vi "CLD 2 Elapsed Time Express FGV Exercise.vi"(7 "Express Timer FGV Enum":enum16{"Reset", "Read Status", "Set Auto Reset"}(ring), 8 "error in (no error)":errorcluster, 9 "Auto Reset (F)":bool, 11 "Time Target (s)":dbl=7.0) -> (0 "error out":errorcluster, 2 "Elapsed Time (s)":dbl, 3 "Time Has Elapsed":bool)   [LabVIEW 2025]
doc: "CLD 2 Exercise"
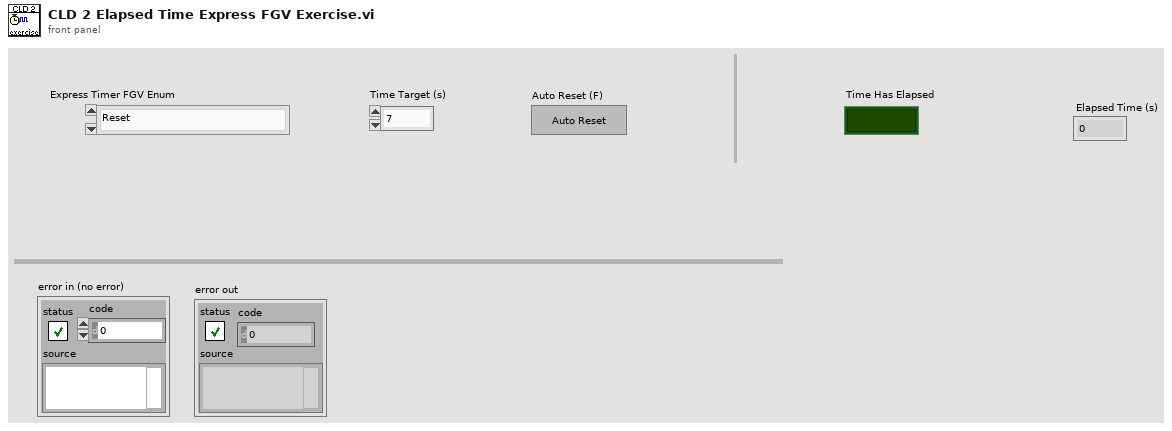
[diagram p1: front panel]
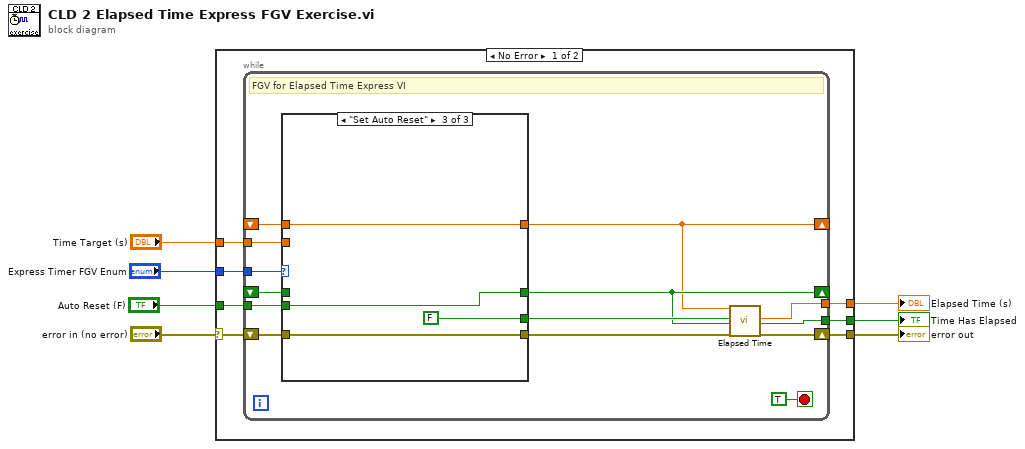
[diagram p0: block diagram]
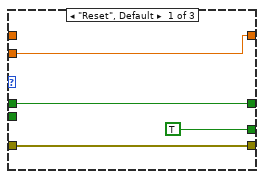
[diagram p2: hidden frame]
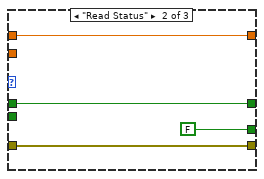
[diagram p3: hidden frame]
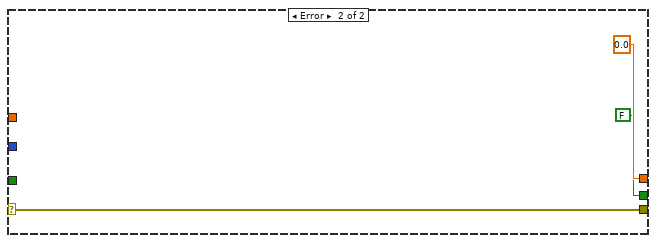
[diagram p4: hidden frame]
diagram:
  n1 = case shown="No Error" "error in (no error)" {
    selector: "error in (no error)" -> [w14 w43]
    tunnel: [w13 w43] -> w6
    tunnel: "Express Timer FGV Enum" -> [w12 _]
    tunnel: [w10 0.0 ("Elapsed Time (s)")] -> w4
    tunnel: [w11 FALSE ("Time has Elapsed")] -> w3
    tunnel: "Time Target (s)" -> [w9 _]
    tunnel: "Auto Reset (F)" -> [w8 _]
    frame No Error {
      n2 = while {
        shift-right: [w22] -> w13
        shift-left: w14 -> [w28]
        tunnel: w12 -> [w25]
        tunnel: [w21] -> w11
        shift-right: [w19] -> _
        shift-left: _ -> [w23]
        shift-right: [w18] -> _
        shift-left: _ -> [w24]
        tunnel: [w17] -> w10
        tunnel: w9 -> [w16]
        tunnel: w8 -> [w15]
        stop <- TRUE stop-if-true
        # "FGV for Elapsed Time Express VI"
        n3 = case shown="\"Set Auto Reset\"" w25 {
          tunnel: w28 -> [w32 w36 w40]
          tunnel: [w32 w36 w40] -> w27
          tunnel: [TRUE FALSE FALSE] -> w20
          tunnel: w24 -> [_ w34 w38]
          tunnel: w23 -> [w30 w35 _]
          tunnel: [w30 w35 w37] -> w19
          tunnel: [w29 w34 w38] -> w18
          tunnel: w16 -> [w29 _ _]
          tunnel: w15 -> [_ _ w37]
          frame "Reset", Default {
          }
          frame "Read Status" {
          }
          frame "Set Auto Reset" {
          }
        }
        n4 = call "Elapsed Time"("Time Target (s)"=w18, "Reset"=w20, "Auto Reset"=w19, "error in (no error)"=w27) -> ("Elapsed Time (s)"=w17:dbl, "Time has Elapsed"=w21:bool, "error out"=w22:errorcluster)  [unwired: 8 in, 5 out]
      }
    }
    frame Error {
    }
  }
  "error out" <- w6
  "Elapsed Time (s)" <- w4
  "Time Has Elapsed" <- w3
